vi "Libary Persist Position and Controls.vi"(0 "action":enum16{"save", "load"}(ring), 1 "do not open (false)":bool, 5 "do not persist bounds (false)":bool, 7 "filename (<window title hash>.dat)":string, 9 "selection regexp ((persistent))":string="(persistent)", 11 "error in (no error)":errorcluster) -> (4 "missing data items? {load}":bool, 15 "error out":errorcluster)   [LabVIEW 2012]
doc: "Persist the content of selected controls on the caller's front panel and optionally persist the panel's position and size (if resizable). The persistence file is stored in the \"persistence data\" subdirectory of default data directory. When the persistence path global is set, a further subdirectory thereof is used. The subset of selected controls is determined by the presence of a specific word or pattern (specified via the \"selection regexp\" input) in the description of the control.\nThe saved data format consist of an array of clusters containing a string set to the name of the control as well as the variant value of the control. When loading the data, the selected controls are initialized with the clusters tagged with their name. This allows for storage of any datatype, and makes the procedure insensitive to reordering of the control tabbing order. When fewer receiving controls are present than stored data items, no error is generated. When no data item could be matched to one or more receiving controls, a descriptive error is generated. You may wish to ignore this error based on its error code as it might be induced after an intended extension of the selected set of controls on your front panel."
uses:
  glb_Library Configuration Globals.vi
panel:
  out "winbounds":T1
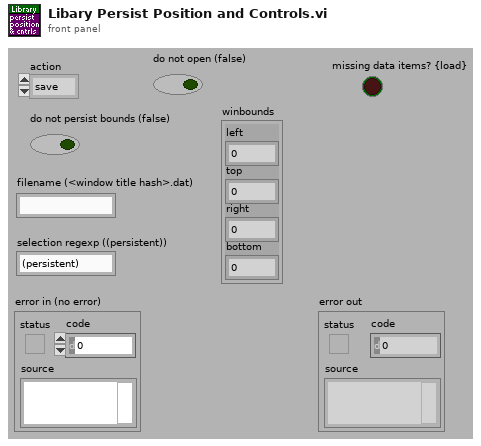
[diagram p1: front panel]
types:
  T1 = cluster{"left":i16, "top":i16, "right":i16, "bottom":i16}
  T2 = typedef "LVRectTypeDef.ctl" = cluster{"Left":i16, "Top":i16, "Right":i16, "Bottom":i16}
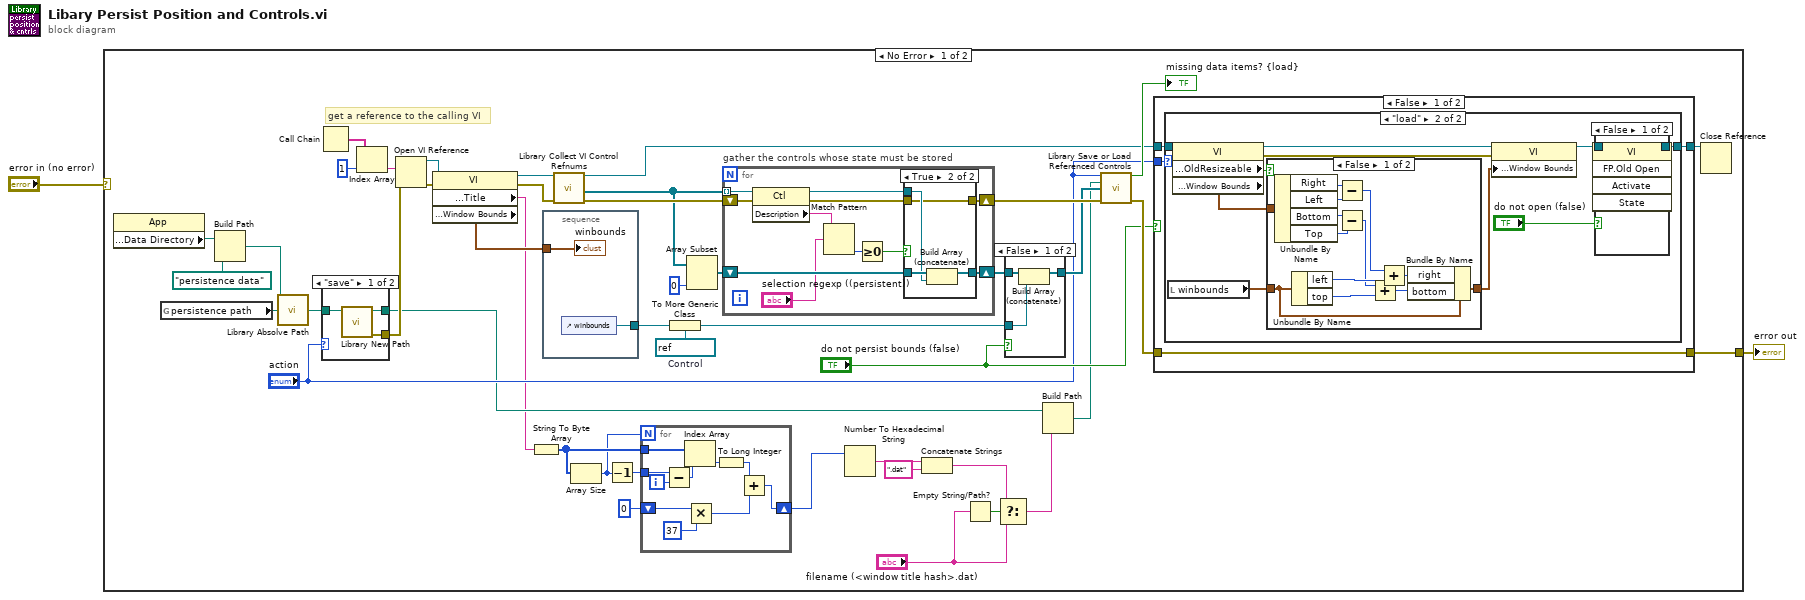
[diagram p0: block diagram]
diagram:
  n1 = case shown="No Error" "error in (no error)" {
    selector: "error in (no error)" -> [_ w119]
    tunnel: [w19 w119] -> w1
    frame No Error {
      w26 = refnum<vi> refnum  # Control
      # "get a reference to the calling VI"
      n2 = property class="App"() -> ("Application:Default:Data Directory"=w3:path)  [unwired: 2 in, 2 out]
      n3 = global read "glb_Library Configuration Globals.vi" "persistence path"() -> (w13:path)
      n4 = Build Path(base path=w3, name or relative path=path "persistence data" ("path in")) -> (appended path=w14:path)
      n5 = call "Library Absolve Path.vi"("absolute base"=w14, "input path to absolve"=w13) -> ("absolved path"=w12:path)  [unwired: 13 in]
      n6 = Call Chain() -> (call chain=w44:string[])
      n7 = case shown="\"save\"" "action" {
        tunnel: [w60 _] -> w17
        tunnel: [w59 w61] -> w16
        tunnel: w12 -> [w58 w61]
        frame "save" {
          n8 = call "Library New Path.vi"("directory path"=w58) -> ("error out"=w60:errorcluster, "dup directory path"=w59:path)  [unwired: 5 in]
        }
        frame "load" {
        }
      }
      n9 = Index Array(array=w44, index=1) -> (element=w42:string)
      n10 = Open VI Reference(vi path=w42, error in (no error)=w17) -> (vi reference=w37:refnum<vi>, error out=w47:errorcluster)  [unwired: 4 in]
      n11 = property class="VI"(reference=w37, error in=w47) -> (reference out=w34:refnum<vi>, error out=w33:errorcluster, "Front Panel Window:Title"=w7:string, "Front Panel Window:Window Bounds"=w30:T2)
      n12 = String To Byte Array(string=w7) -> (unsigned byte array=w10:u8[])
      n13 = stacked-sequence {
        tunnel: w30 -> [w101]
        tunnel: [w100] -> w28
        frame #0 {
          n14 = control-ref of="winbounds"() -> (w100:refnum<vi>)
          "winbounds" <- w101
        }
      }
      n15 = call "Library Collect VI Control Refnums.vi"("VI refnum in"=w34, "error in (no error)"=w33) -> ("VI refnum out"=w24:refnum<vi>, "control refnums"=w31:refnum<vi>[], "error out"=w32:errorcluster)  [unwired: 11 in]
      n16 = Array Size(array=w10) -> (size(s)=w8:i32)
      n17 = Decrement(x=w8) -> (x-1=w9:i32)
      n18 = for {
        N: w8 -> [_]
        shift-right: [w48] -> w6
        shift-left: 0 -> [w52]
        tunnel: w10 -> [w55]
        tunnel: w9 -> [w57]
        i -> [w56]
        n19 = Subtract(x=w57, y=w56) -> (x-y=w54:i32)
        n20 = Index Array(array=w55, index=w54) -> (element=w51:u8)
        n21 = Multiply(x=w52, y=37 ("x")) -> (x*y=w50:i32)
        n22 = To Long Integer(number=w51) -> (32bit integer=w49:i32)
        n23 = Add(x=w49, y=w50) -> (x+y=w48:i32)
      }
      n24 = To More Generic Class(target class=w26, reference=w28) -> (generic class reference=w27:refnum<vi>)
      n25 = Array Subset(array=w31, length=0 ("Array Length")) -> (w46:refnum<vi>[])  [unwired: 1 in]
      n26 = for "gather the controls whose state must be stored" {
        tunnel: w31 -> [w107] mode=indexing
        shift-right: [w108] -> w41
        shift-left: w46 -> [w109]
        shift-right: [w102] -> w36
        shift-left: w32 -> [w104]
        n27 = property class="Ctl"(reference=w107, error in=w104) -> (reference out=w106:refnum<vi>, error out=w103:errorcluster, "Description"=w112:string)
        n28 = Match Pattern(string=w112, regular expression="selection regexp ((persistent))") -> (offset past match=w111:i32)  [unwired: 1 in, 3 out]
        n29 = Greater Or Equal To 0?(x=w111) -> (x >= 0?=w110:bool)
        n30 = case shown="True" w110 {
          tunnel: w109 -> [w114 w118]
          tunnel: [w114 w117] -> w108
          tunnel: w106 -> [_ w116]
          tunnel: w103 -> [w113 w115]
          tunnel: [w113 w115] -> w102
          frame False {
          }
          frame True {
            n31 = Build Array (concatenate)(w118, w116) -> (w117:refnum<vi>[])
          }
        }
      }
      n32 = Number To Hexadecimal String(2:w6) -> (0:w5:string)  [unwired: 1 in]
      n33 = Concatenate Strings(w5, ".dat" ("string")) -> (w21:string)
      n34 = Empty String/Path?(string/path="filename (<window title hash>.dat)") -> (empty?=w40:bool)
      n35 = Select(t=w21, s=w40, f="filename (<window title hash>.dat)") -> (s? t:f=w38:string)
      n36 = case shown="False" "do not persist bounds (false)" {
        tunnel: w41 -> [w98 w99]
        tunnel: [w97 w99] -> w29
        tunnel: w27 -> [w96 _]
        frame False {
          n37 = Build Array (concatenate)(w98, w96) -> (w97:refnum<vi>[])
        }
        frame True {
        }
      }
      n38 = Build Path(base path=w16, name or relative path=w38) -> (appended path=w18:path)
      n39 = call "Library Save or Load Referenced Controls.vi"("action"="action", "file path"=w18, "control refs"=w29, "error in (no error)"=w36) -> ("missing data items? {load}"=→"missing data items? {load}":bool, "error out"=w25:errorcluster)  [unwired: 8 in, 2 out]
      n40 = case shown="False" "do not persist bounds (false)" {
        tunnel: w25 -> [w62 w95]
        tunnel: [w62 w95] -> w19
        tunnel: [w64 w94] -> w23
        tunnel: w24 -> [w65 w94]
        tunnel: "action" -> [w63 _]
        frame False {
          n41 = case shown="\"load\"" w63 {
            tunnel: w65 -> [w66 w76]
            tunnel: [w66 w68] -> w64
            frame "save" {
            }
            frame "load" {
              n42 = local read "winbounds"() -> (w71:T1)
              n43 = property class="VI"(reference=w76) -> (reference out=w75:refnum<vi>, error out=w74:errorcluster, "Front Panel Window:OldResizeable"=w73:bool, "Front Panel Window:Window Bounds"=w72:T2)  [unwired: 1 in]
              n44 = case shown="False" w73 {
                tunnel: w72 -> [w92 _]
                tunnel: w71 -> [w83 w93]
                tunnel: [w80 w93] -> w70
                frame False {
                  n45 = Unbundle By Name(w92) -> ("Right"=w91:i16, "Left"=w90:i16, "Bottom"=w89:i16, "Top"=w88:i16)
                  n46 = Unbundle By Name(w83) -> ("left"=w86:i16, "top"=w84:i16)
                  n47 = Subtract(x=w91, y=w90) -> (x-y=w87:i16)
                  n48 = Subtract(x=w89, y=w88) -> (x-y=w85:i16)
                  n49 = Add(x=w85, y=w84) -> (x+y=w81:i16)
                  n50 = Add(x=w87, y=w86) -> (x+y=w82:i16)
                  n51 = Bundle By Name(cluster=w83, "right"=w82, "bottom"=w81) -> (w80:T1)
                }
                frame True {
                }
              }
              n52 = property class="VI"(reference=w75, error in=w74, "Front Panel Window:Window Bounds"=w70) -> (reference out=w69:refnum<vi>)  [unwired: 1 out]
              n53 = case shown="False" "do not open (false)" {
                tunnel: w69 -> [w78 w79]
                tunnel: [w77 w79] -> w68
                frame False {
                  n54 = invoke class="VI" method="FP.Old Open"(reference=w78) -> (reference out=w77:refnum<vi>)  [unwired: 4 in, 4 out]
                }
                frame True {
                }
              }
            }
          }
        }
        frame True {
        }
      }
      n55 = Close Reference(reference=w23) -> ()  [unwired: 1 in, 1 out]
    }
    frame Error {
    }
  }
  "error out" <- w1
